vi "Panel.vi"(6 "Fiber Auto Collimation state data":refnum<class "Fiber Auto Collimation state data.lvclass">, 7 "Station config":refnum<class "Station config.lvclass">, 8 "error in":errorcluster, 11 "Fiber Auto Collimation configuration panel in":refnum<class "Fiber Auto Collimation configuration panel.lvclass">) -> (0 "error out":errorcluster, 3 "Fiber Auto Collimation configuration panel out":refnum<class "Fiber Auto Collimation configuration panel.lvclass">)   [LabVIEW 2018, in "Fiber Auto Collimation configuration panel.lvclass"]
doc: "This is the configuration panel. It is designed both as a starter location for all station administration controls and also to potentially be used as a template for copying to start off other Panel classes used on stations as well."
uses:
  Fiber Auto Collimation configuration panel.lvclass
  C:/LabVIEW Code/Fiber Auto Collimation/Source/Panels/Fiber Auto Collimation panel.lvclass
  State data/Fiber Auto Collimation state data.lvclass
  <userlib>/Recipe/Station Config/Station config.lvclass
  State data/Tracked state data.ctl
  State data/Fiber Auto Collimation state data.lvclass/Fiber Auto Collimation state data.ctl
  403c9101-8a94-4915-b1d2-c2bcb50c0ac3.vi
  14963872-09c7-484d-8f8b-814a5689ce7f.vi
  f712ade7-1d53-4238-a979-a732add69fae.vi
  403c9101-8a94-4915-b1d2-c2bcb50c0ac3.vi/f33612d2-cbd2-4a12-8b29-77b7af87b990.vi
  <userlib>/nLight Tidbits/Misc/Convert True to Enabled.vi
  <userlib>/nLight Error Handling/Log any errors.vi
  References/Obtain control updates queue.vi
  Misc SubVIs/Get control name.vi
  <userlib>/nLight Error Handling/Merge errors no loss.vi
  <userlib>/Recipe/Test Recipe classes/Test Recipe.lvclass
  ee343da0-43c2-4897-a8b1-c706a9c51c79.vi
  a23b397d-d5c1-4275-a046-494f1c6e56ee.vi
  References/Fiber Auto Collimation References.lvclass
  Fiber Auto Collimation panel.lvclass
panel:
  out "Loaded test recipe name":string
  in  "Upload test recipe":bool
  in  "Edit test recipe":bool
  in  "Edit test recipe keys":bool
  in  "Basic station config":bool
  in  "Edit station config keys":bool
  in  "Configure instruments":bool
  in  "Upload station config":bool
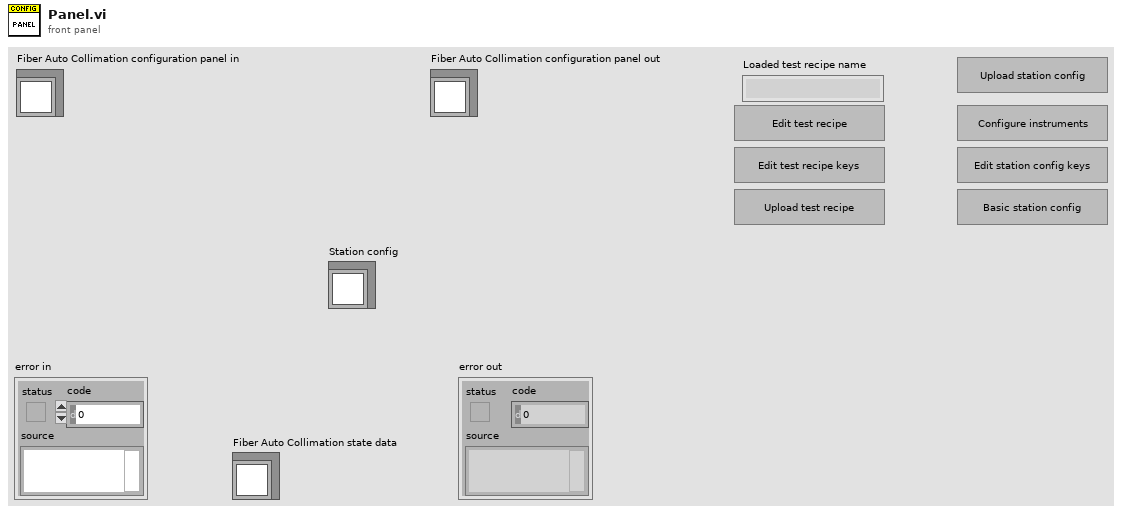
[diagram p1: front panel]
types:
  T1 = typedef "Fiber Auto Collimation state data.lvclass/Tracked state data.ctl" = enum16{"No update", "Permission level", "Username", "Test running", "DUT Serial", "Test status", "MOM Lot", "Loaded test recipe", "Model case running", "Station status", "BV data", "Defect Identify data", "Axis Position data", "Fiber Ass PN", "Operator", "RunTime", "VBAI", "Steps Cycle Time"}
  T2 = cluster{"事件注册引用句柄":refnum<event-registration>, "事件注册引用句柄":refnum<event-registration>}
  T3 = enum8{"Enabled", "Disabled", "Disabled and Grayed Out"}
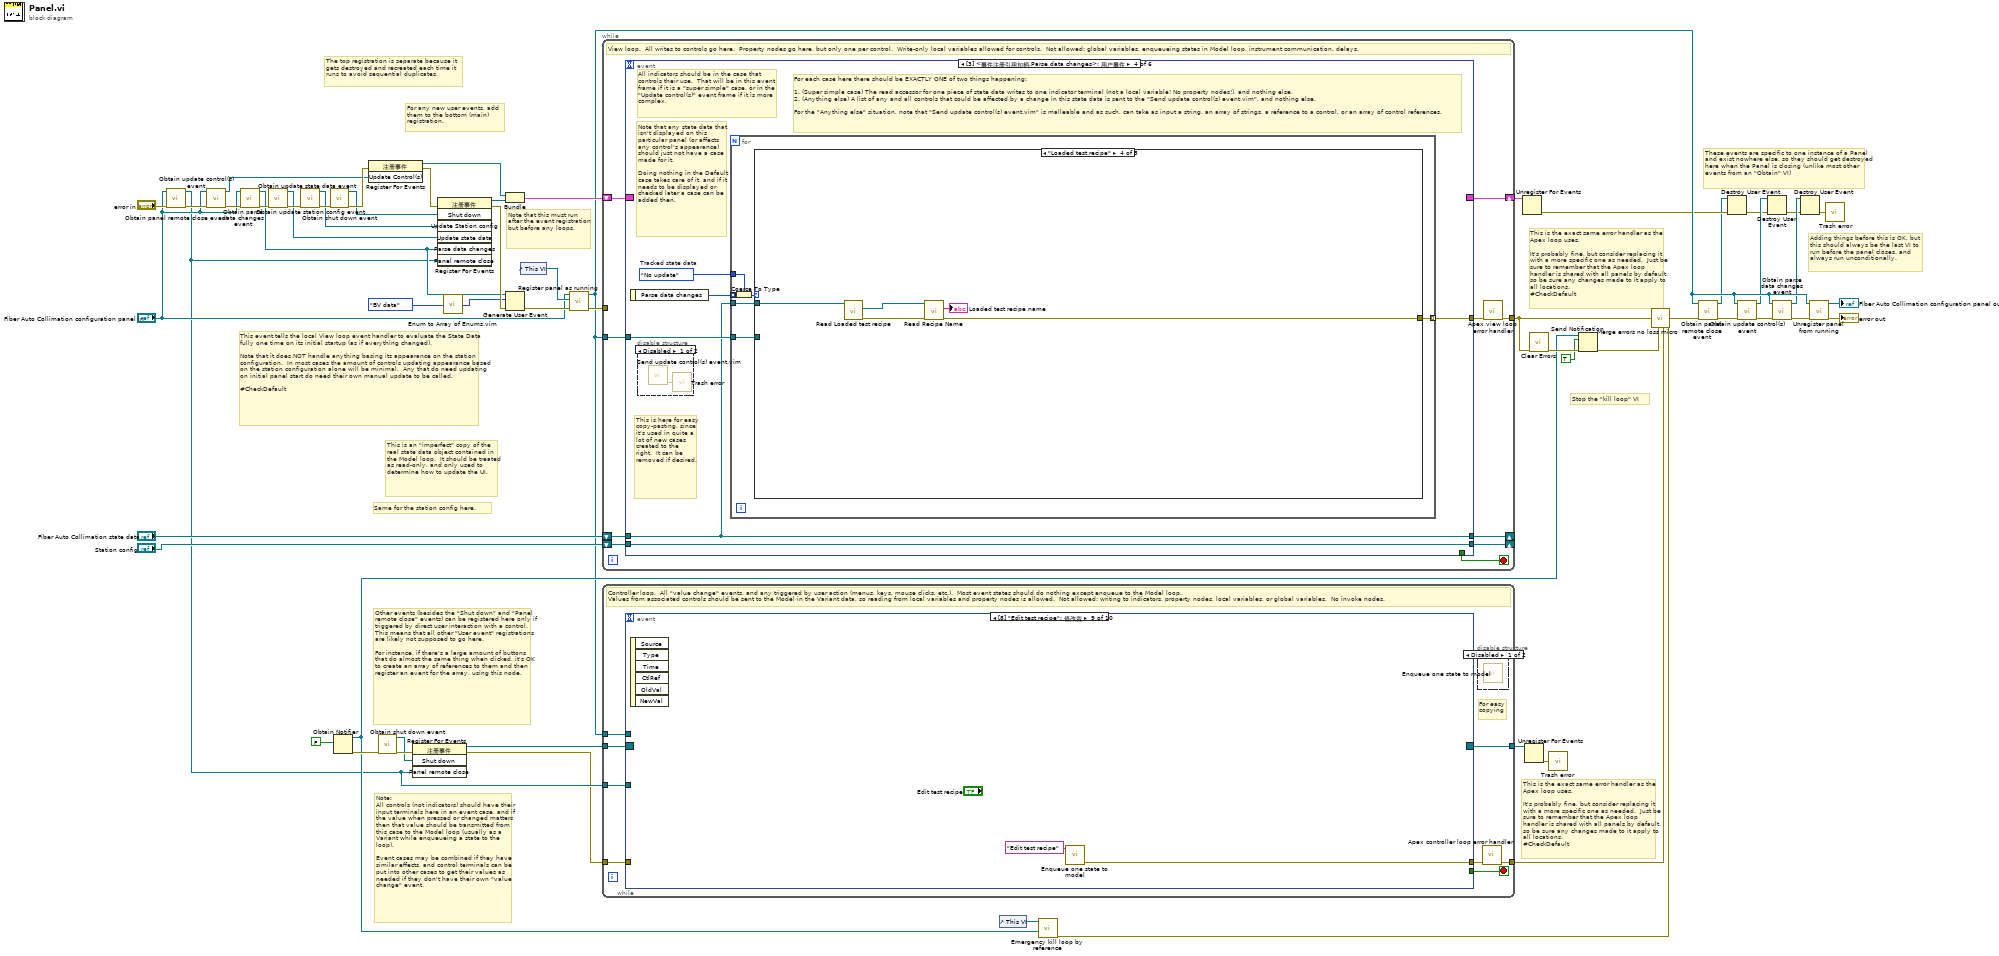
[diagram p0: block diagram]
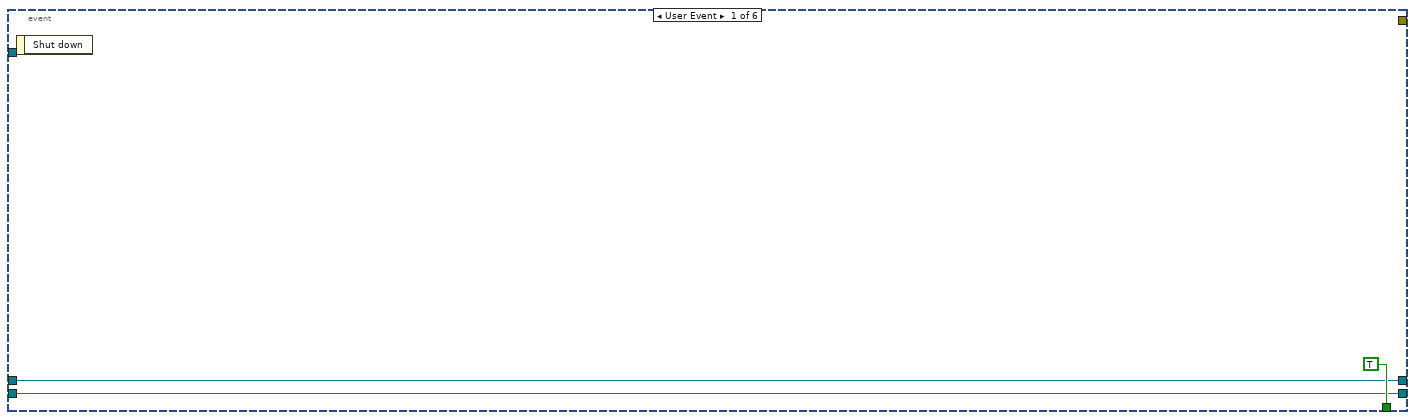
[diagram p2: hidden frame]
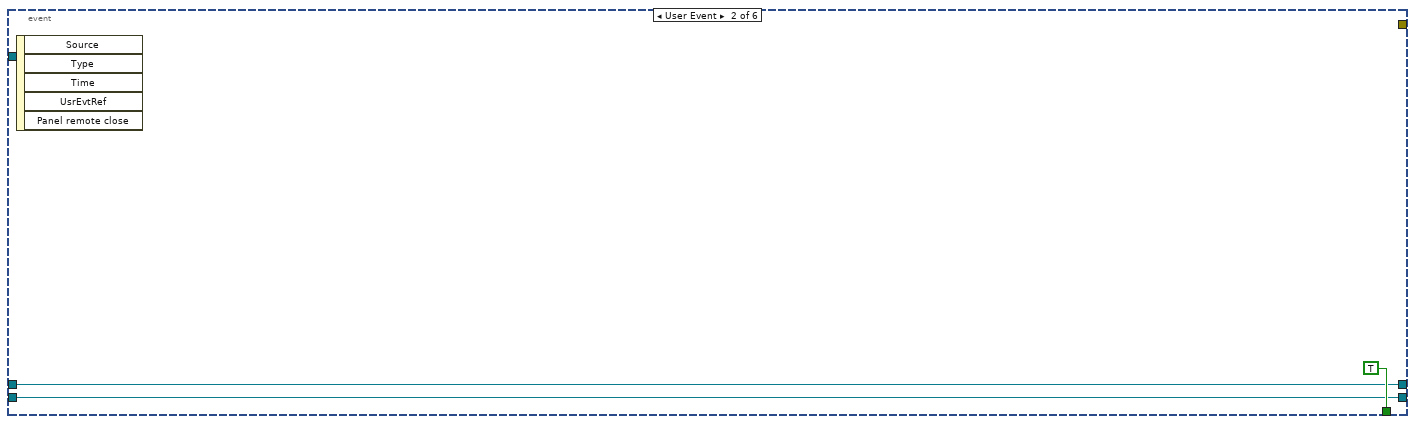
[diagram p3: hidden frame]
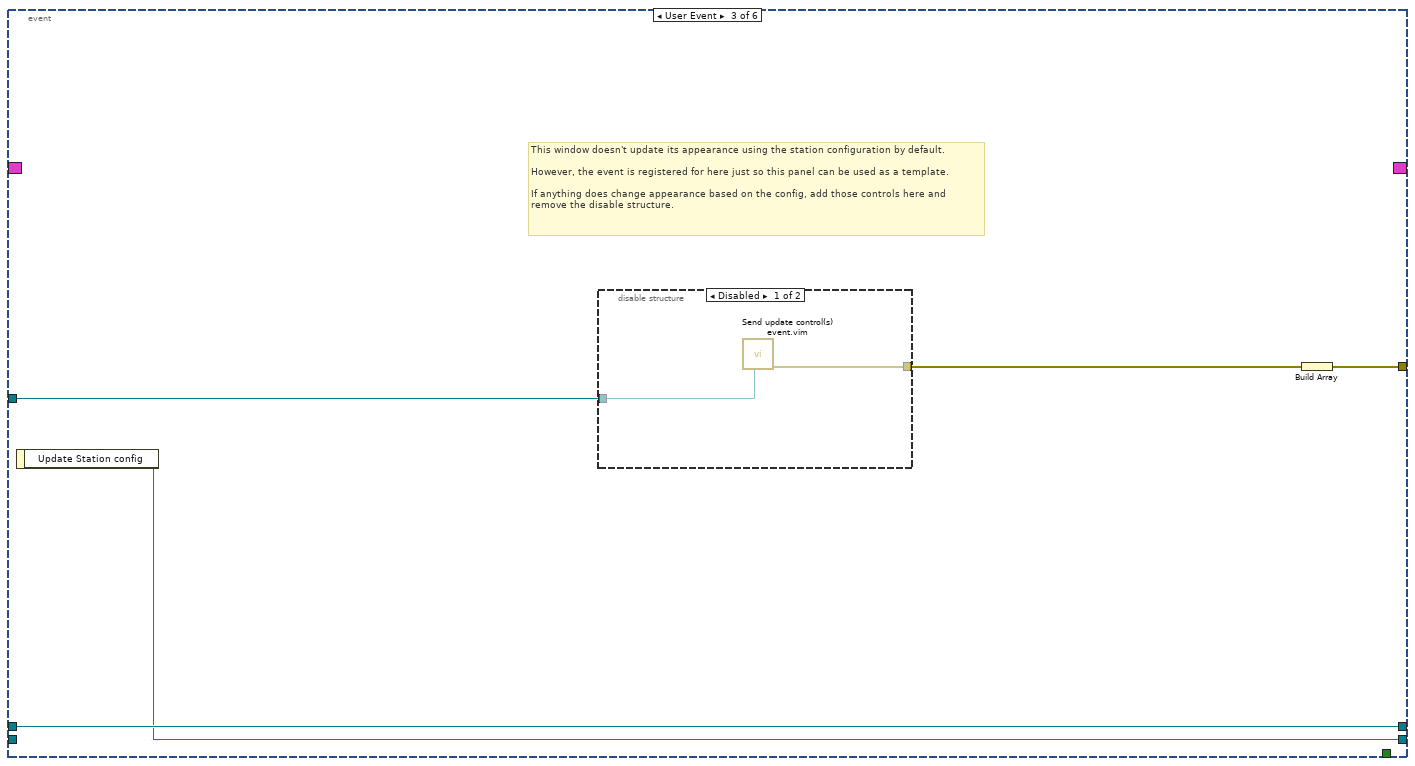
[diagram p4: hidden frame]
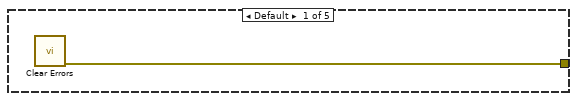
[diagram p7: hidden frame]
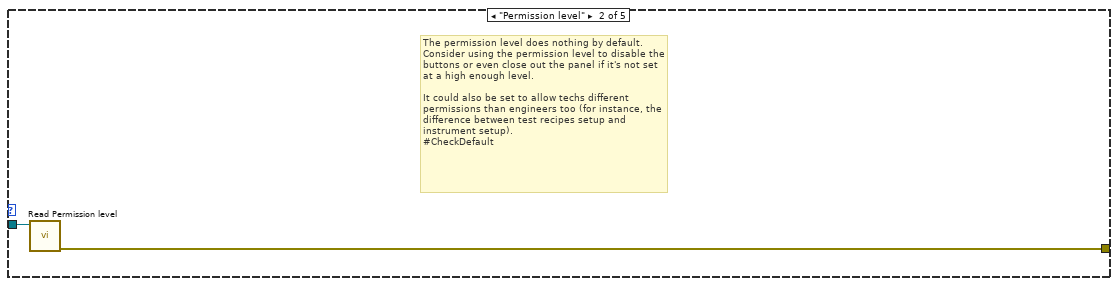
[diagram p8: hidden frame]
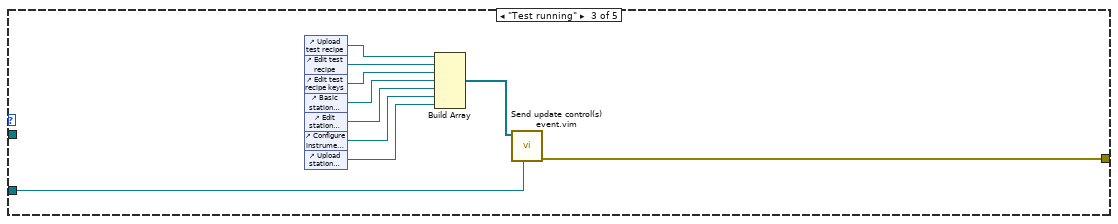
[diagram p9: hidden frame]
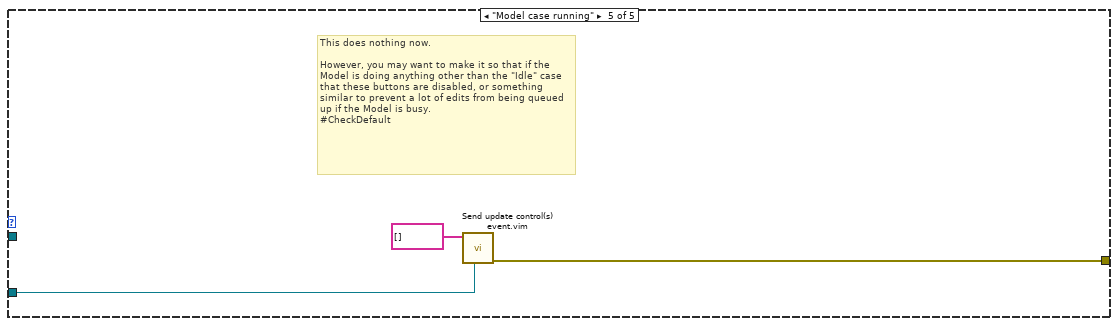
[diagram p10: hidden frame]
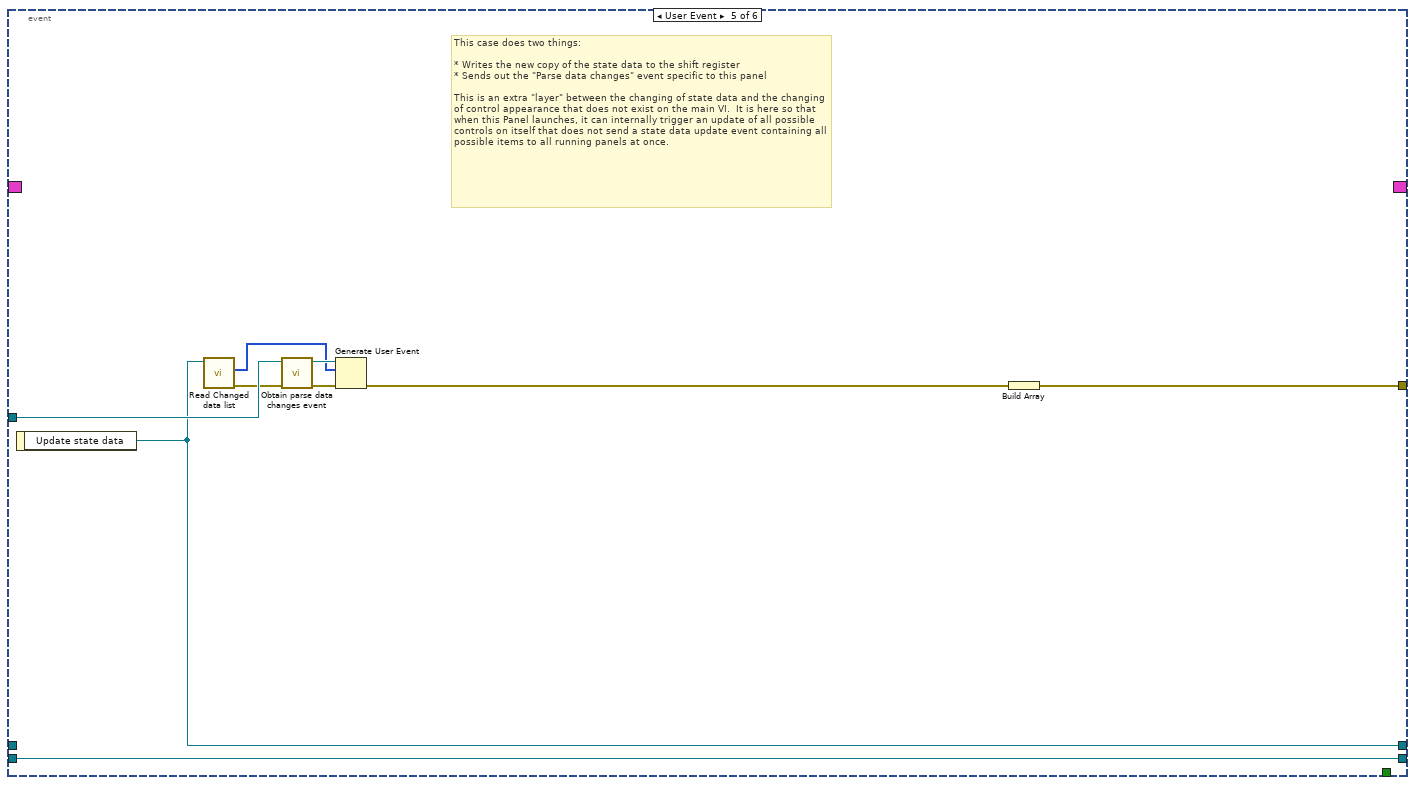
[diagram p11: hidden frame]
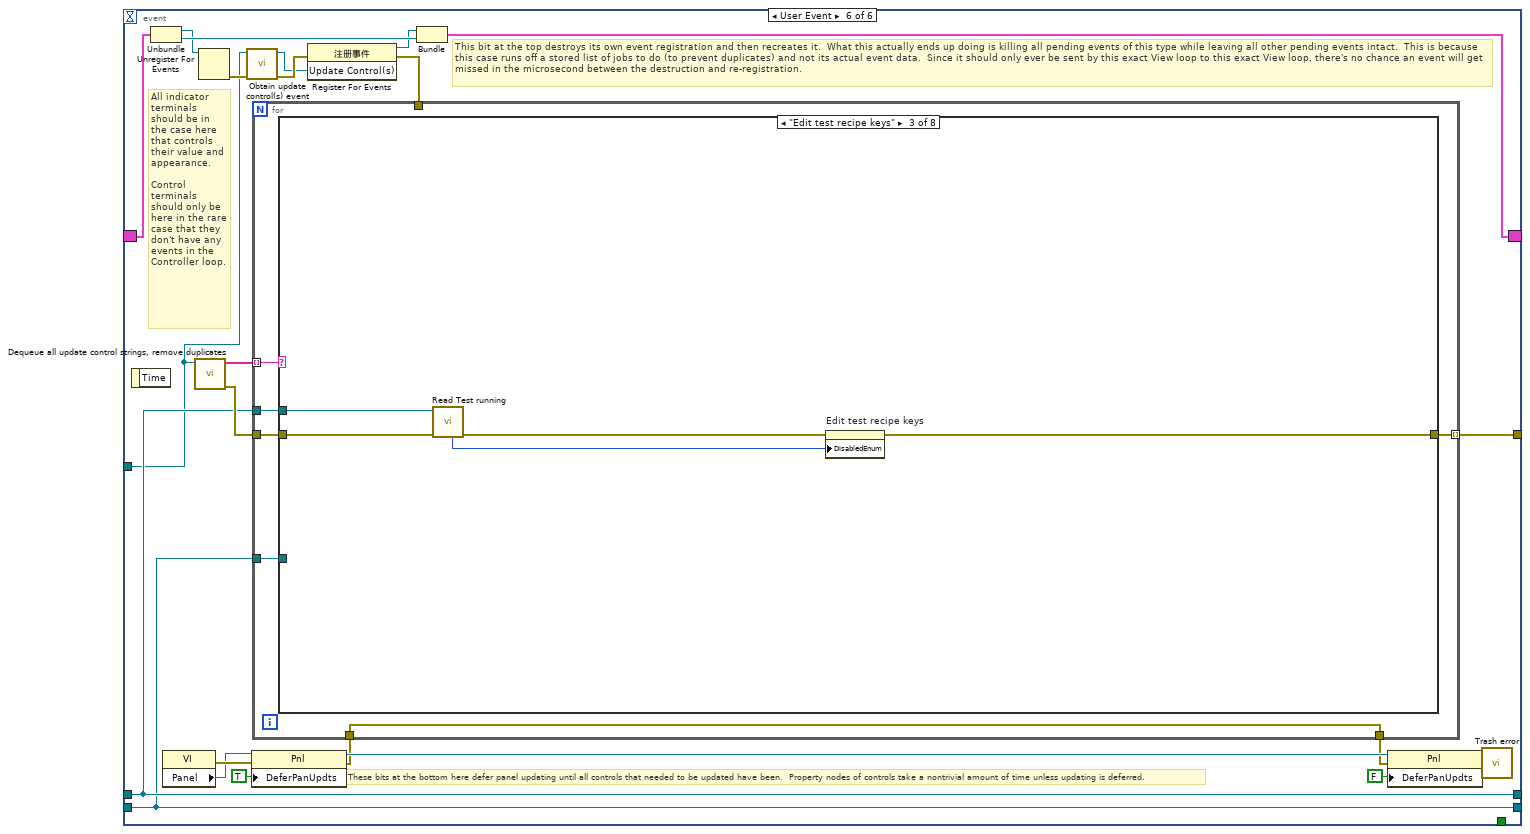
[diagram p12: hidden frame]
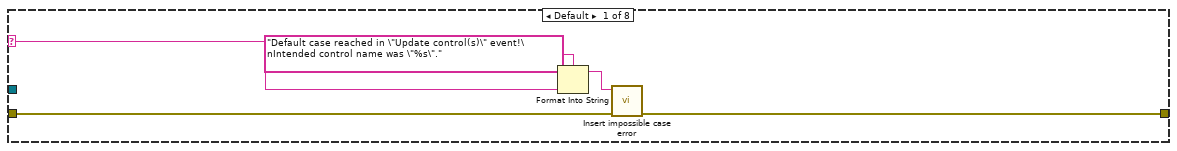
[diagram p13: hidden frame]
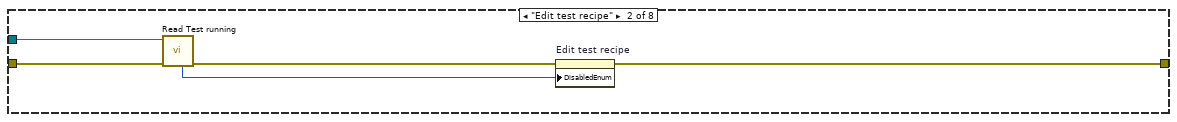
[diagram p14: hidden frame]
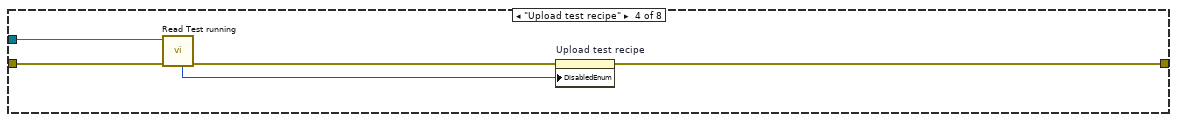
[diagram p15: hidden frame]
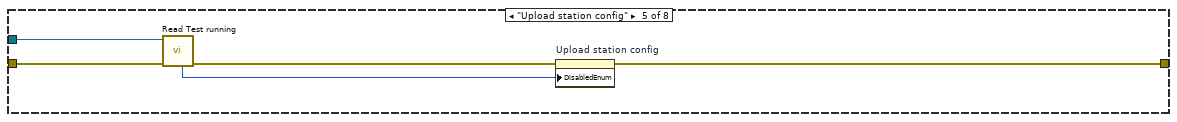
[diagram p16: hidden frame]
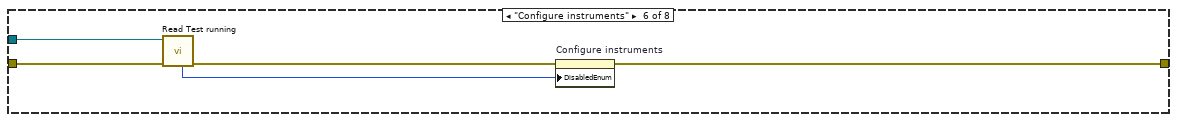
[diagram p17: hidden frame]
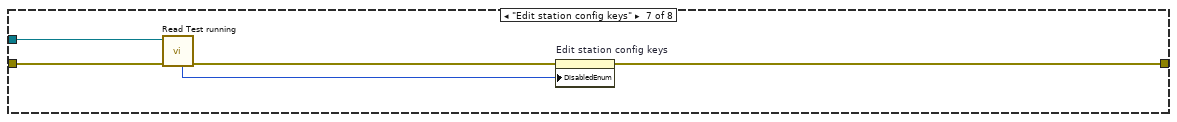
[diagram p18: hidden frame]
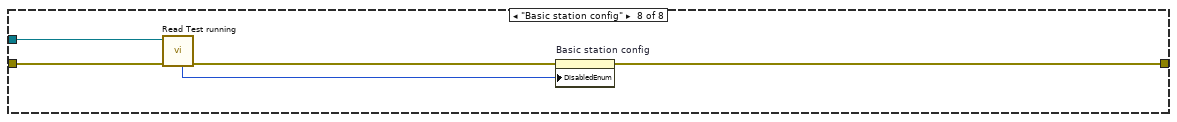
[diagram p19: hidden frame]
diagram:
  # "These events are specific to one instance of a Panel and exist nowhere else, so they should get destroyed here when the Panel is closing (unlike most other events from an \"Obtain\" VI)"
  # "This is the exact same error handler as the Apex loop uses.\n\nIt's probably fine, but consider replacing it with a more specific one as needed.  Just be sure to remember that the Apex loop handler is shared with all panels by default, so be sure any changes made to it apply to all locations.\n#CheckDefault"
  # "Note that this must run after the event registration but before any loops."
  # "This is the exact same error handler as the Apex loop uses.\n\nIt's probably fine, but consider replacing it with a more specific one as needed.  Just be sure to remember that the Apex loop handler is shared with all panels by default, so be sure any changes made to it apply to all locations.\n#CheckDefault"
  # "This event tells the local View loop event handler to evaluate the State Data fully one time on its initial startup (as if everything changed).\n\nNote that it does NOT handle anything basing its appearance on the station configuration.  In most cases the amount of controls updating appearance based on the station configuration alone will be minimal.  Any that do need updating on initial panel start do need their own manual update to be called.\n\n#CheckDefault"
  # "Adding things before this is OK, but this should always be the last VI to run before the panel closes, and always run unconditionally."
  # "Stop the \"kill loop\" VI"
  # "Same for the station config here."
  # "Note:\nAll controls (not indicators) should have their input terminals here in an event case, and if the value when pressed or changed matters then that value should be transmitted from this case to the Model loop (usually as a Variant while enqueueing a state to the loop).\n\nEvent cases may be combined if they have similar effects, and control terminals can be put into other cases to get their values as needed if they don't have their own \"value change\" event."
  # "Other events (besides the \"Shut down\" and \"Panel remote close\" events) can be registered here only if triggered by direct user interaction with a control.  This means that all other \"User event\" registrations are likely not supposed to go here.\n\nFor instance, if there's a large amount of buttons that do almost the same thing when clicked, it's OK to create an array of references to them and then register an event for the array, using this node."
  # "For any new user events, add them to the bottom (main) registration."
  # "The top registration is separate because it gets destroyed and recreated each time it runs to avoid sequential duplicates."
  # "This is an \"imperfect\" copy of the real state data object contained in the Model loop.  It should be treated as read-only, and only used to determine how to update the UI."
  n1 = call "Obtain panel remote close event.vi"("error in (no error)"="error in", "Fiber Auto Collimation panel"="Fiber Auto Collimation configuration panel in") -> ("error out"=w56:errorcluster, "Panel remote close"=w17:refnum<user-event>)  [unwired: 8 in]
  n2 = call "Obtain update control(s) event.vi"("error in (no error)"=w56, "Fiber Auto Collimation panel"="Fiber Auto Collimation configuration panel in") -> ("error out"=w27:errorcluster, "Update Control(s)"=w45:refnum<user-event>)  [unwired: 8 in]
  n3 = call "Obtain parse data changes event.vi"("error in (no error)"=w27, "Fiber Auto Collimation panel"="Fiber Auto Collimation configuration panel in") -> ("error out"=w26:errorcluster, "Parse data changes"=w24:refnum<user-event>)  [unwired: 8 in]
  n4 = call "Obtain update state data event.vi"("error in (no error)"=w26) -> ("error out"=w54:errorcluster, "Update state data"=w47:refnum<user-event>)  [unwired: 9 in]
  n5 = call "Obtain update station config event.vi"("error in"=w54) -> ("error out"=w49:errorcluster, "Update Station config"=w48:refnum<user-event>)  [unwired: 9 in]
  n6 = call "Obtain shut down event.vi"("error in (no error)"=w49) -> ("error out"=w57:errorcluster, "Shut down"=w53:refnum<user-event>)  [unwired: 9 in]
  n7 = Obtain Notifier(notification data type=FALSE) -> (notifier out=w38:refnum<notifier>, error out=w41:errorcluster)  [unwired: 3 in, 1 out]
  n8 = register-events(error in=w57, w45) -> (reference out=w44:refnum<event-registration>, error out=w32:errorcluster)  [unwired: 1 in]
  n9 = call "Obtain shut down event.vi"("error in (no error)"=w41) -> ("error out"=w52:errorcluster, "Shut down"=w51:refnum<user-event>)  [unwired: 9 in]
  n10 = register-events(error in=w52, w51, w17) -> (reference out=w50:refnum<event-registration>, error out=w1:errorcluster)  [unwired: 1 in]
  n11 = register-events(error in=w32, w53, w48, w47, w24, w17) -> (reference out=w46:refnum<event-registration>, error out=w55:errorcluster)  [unwired: 1 in]
  n12 = call "Enum to Array of Enums.vim"("enum"=Tracked_state_data."BV data" ("Tracked state data")) -> ("array of enums"=w23:T1[])
  n13 = Bundle("事件注册引用句柄"=w44, "事件注册引用句柄"=w46) -> (w43:T2)  [unwired: 1 in]
  n14 = Generate User Event(user event=w24, event data cluster=w23, error in=w55) -> (error out=w21:errorcluster)  [unwired: 1 in, 1 out]
  n15 = control-ref of="This VI"() -> (w31:refnum<vi>)
  n16 = call "Register panel as running.vi"("error in (no error)"=w21, "\"This VI\" reference from current panel"=w31, "Fiber Auto Collimation panel in"="Fiber Auto Collimation configuration panel in") -> ("error out"=w22:errorcluster, "Fiber Auto Collimation panel out"=w10:refnum<class "Fiber Auto Collimation configuration panel.lvclass">)  [unwired: 7 in]
  n17 = while {
    tunnel: [w67] -> w34
    shift-right: [w63] -> _
    shift-left: "Fiber Auto Collimation state data" -> [w62]
    shift-right: [w61] -> w16
    shift-left: w43 -> [w66]
    shift-right: [w60] -> _
    shift-left: "Station config" -> [w59]
    tunnel: w10 -> [w58]
    tunnel: w22 -> [_]
    stop <- w64 stop-if-true
    # "View loop.  All writes to controls go here.  Property nodes go here, but only one per control.  Write-only local variables allowed for controls.  Not allowed: global variables, enqueueing states in Model loop, instrument communication, delays."
    n18 = event "View" shown="[3] <事件注册引用句柄.Parse data changes>: 用户事件" {
      selector: w66 -> [_ _ _ _ _ w146]
      dyn-events: [_ _ _ _ _ w139] -> w61
      timeout: _ -> [_ _ _ _ _ _]
      tunnel: [_ _ w75 w86 w120 w128] -> w65
      tunnel: [TRUE TRUE _ _ _ _] -> w64
      tunnel: [w69 w72 w78 w83 w117 w129] -> w63
      tunnel: w62 -> [w69 w72 w78 w83 _ w129]
      tunnel: [w68 w71 w77 w85 w123 w126] -> w60
      tunnel: w59 -> [w68 w71 _ w85 w123 w126]
      tunnel: w58 -> [_ _ w74 w84 w122 w125]
      event User Event {
        n19 = event-data() -> ()  [unwired: 1 in, 1 out]
      }
      event User Event {
        n20 = event-data() -> ()  [unwired: 1 in, 5 out]
      }
      event User Event {
        # "This window doesn't update its appearance using the station configuration by default.\n\nHowever, the event is registered for here just so this panel can be used as a template.\n\nIf anything does change appearance based on the config, add those controls here and  remove the disable structure."
        n21 = event-data() -> ("Update Station config"=w77:refnum<class "Station config.lvclass">)  [unwired: 1 in]
        n22 = disable-structure shown="Disabled" {
          disable-tunnel: [w80 _] -> w76
          disable-tunnel: w74 -> [w79 _]
          frame Disabled {
            n23 = call "Send update control(s) event.vim"("Fiber Auto Collimation panel"=w79) -> ("error out"=w80:errorcluster)  [unwired: 10 in]
          }
          frame Enabled {
          }
        }
        n24 = Build Array(w76) -> (w75:errorcluster[])
      }
      event User Event {
        w81 = Tracked_state_data."No update"  # Tracked state data
        # "Note that any state data that isn't displayed on this particular panel (or affects any control's appearance) should just not have a case made for it.  \n\nDoing nothing in the Default case takes care of it, and if it needs to be displayed or checked later a case can be added then."
        # "All indicators should be in the case that controls their use.  That will be in this event frame if it is a \"super simple\" case, or in the \"Update control(s)\" event frame if it is more complex."
        # "This is here for easy copy-pasting, since it's used in quite a lot of new cases created to the right.  It can be removed if desired."
        # "For each case here there should be EXACTLY ONE of two things happening:\n\n1. (Super simple case) The read accessor for one piece of state data writes to one indicator terminal (not a local variable! No property nodes!), and nothing else.\n2. (Anything else) A list of any and all controls that could be affected by a change in this state data is sent to the \"Send update control(s) event.vim\", and nothing else.\n\nFor the \"Anything else\" situation, note that \"Send update control(s) event.vim\" is malleable and as such, can take as input a string, an array of strings, a reference to a control, or an array of control references."
        n25 = event-data() -> ("Parse data changes"=w82:u16[])  [unwired: 1 in]
        n26 = disable-structure shown="Disabled" {
          frame Disabled {
            n27 = call "Send update control(s) event.vim"() -> ("error out"=w87:errorcluster)  [unwired: 11 in]
            n28 = call <userlib>:"Trash error.vi"("error in"=w87) -> ()  [unwired: 15 in]
          }
          frame Enabled {
          }
        }
        n29 = for {
          tunnel: w82 -> [w93] mode=indexing
          tunnel: w83 -> [w92]
          tunnel: [w91] -> w86 mode=indexing
          tunnel: w84 -> [w90]
          tunnel: w81 -> [w88]
          n30 = Coerce To Type(0:w93, 1:w88) -> (2:w89:T1)
          n31 = case shown="\"Loaded test recipe\"" w89 {
            tunnel: w92 -> [_ w96 _ w111 _]
            tunnel: [w94 w95 w106 w108 w114] -> w91
            tunnel: w90 -> [_ _ w105 _ w112]
            frame Default {
              n32 = call <vilib>:"Clear Errors.vi"() -> ("error out"=w94:errorcluster)  [unwired: 6 in, 1 out]
            }
            frame "Permission level" {
              # "The permission level does nothing by default.  Consider using the permission level to disable the buttons or even close out the panel if it's not set at a high enough level.  \n\nIt could also be set to allow techs different permissions than engineers too (for instance, the difference between test recipes setup and instrument setup).\n#CheckDefault"
              n33 = call "Read Permission level.vi"("Fiber Auto Collimation state data in"=w96) -> ("error out"=w95:errorcluster)  [unwired: 8 in, 2 out]
            }
            frame "Test running" {
              n34 = control-ref of="Upload test recipe"() -> (w104:refnum<vi>)
              n35 = control-ref of="Edit test recipe"() -> (w103:refnum<vi>)
              n36 = control-ref of="Edit test recipe keys"() -> (w102:refnum<vi>)
              n37 = control-ref of="Basic station config"() -> (w101:refnum<vi>)
              n38 = control-ref of="Edit station config keys"() -> (w100:refnum<vi>)
              n39 = control-ref of="Configure instruments"() -> (w99:refnum<vi>)
              n40 = control-ref of="Upload station config"() -> (w98:refnum<vi>)
              n41 = Build Array(w104, w103, w102, w101, w100, w99, w98) -> (w97:refnum<vi>[])
              n42 = call "Send update control(s) event.vim"("Fiber Auto Collimation panel"=w105, "Control(s) [String or reference, can be array]"=w97) -> ("error out"=w106:errorcluster)  [unwired: 9 in]
            }
            frame "Loaded test recipe" {
              n43 = call "Read Loaded test recipe.vi"("Fiber Auto Collimation state data in"=w111) -> ("error out"=w109:errorcluster, "Loaded test recipe"=w110:refnum<class "Test Recipe.lvclass">)  [unwired: 8 in, 1 out]
              n44 = call-dynamic "Read Recipe Name.vi"("error in (no error)"=w109, "nLight Recipe in"=w110) -> ("error out"=w108:errorcluster, "Recipe Name"=→"Loaded test recipe name":string)  [unwired: 7 in, 1 out]
            }
            frame "Model case running" {
              # "This does nothing now.\n\nHowever, you may want to make it so that if the Model is doing anything other than the \"Idle\" case that these buttons are disabled, or something similar to prevent a lot of edits from being queued up if the Model is busy.\n#CheckDefault"
              n45 = call "Send update control(s) event.vim"("Fiber Auto Collimation panel"=w112, "Control(s) [String or reference, can be array]"=string[] []) -> ("error out"=w114:errorcluster)  [unwired: 9 in]
            }
          }
        }
      }
      event User Event {
        # "This case does two things:\n\n* Writes the new copy of the state data to the shift register\n* Sends out the \"Parse data changes\" event specific to this panel\n\nThis is an extra \"layer\" between the changing of state data and the changing of control appearance that does not exist on the main VI.  It is here so that when this Panel launches, it can internally trigger an update of all possible controls on itself that does not send a state data update event containing all possible items to all running panels at once."
        n46 = event-data() -> ("Update state data"=w117:refnum<class "Fiber Auto Collimation state data.lvclass">)  [unwired: 1 in]
        n47 = call "Read Changed data list.vi"("Fiber Auto Collimation state data in"=w117) -> ("error out"=w116:errorcluster, "Changed data list"=w115:T1[])  [unwired: 8 in, 1 out]
        n48 = call "Obtain parse data changes event.vi"("error in (no error)"=w116, "Fiber Auto Collimation panel"=w122) -> ("error out"=w121:errorcluster, "Parse data changes"=w118:refnum<user-event>)  [unwired: 8 in]
        n49 = Generate User Event(user event=w118, event data cluster=w115, error in=w121) -> (error out=w119:errorcluster)  [unwired: 1 in, 1 out]
        n50 = Build Array(w119) -> (w120:errorcluster[])
      }
      event User Event {
        # "All indicator terminals should be in the case here that controls their value and appearance.\n\nControl terminals should only be here in the rare case that they don't have any events in the Controller loop."
        # "These bits at the bottom here defer panel updating until all controls that needed to be updated have been.  Property nodes of controls take a nontrivial amount of time unless updating is deferred."
        # "This bit at the top destroys its own event registration and then recreates it.  What this actually ends up doing is killing all pending events of this type while leaving all other pending events intact.  This is because this case runs off a stored list of jobs to do (to prevent duplicates) and not its actual event data.  Since it should only ever be sent by this exact View loop to this exact View loop, there's no chance an event will get missed in the microsecond between the destruction and re-registration."
        n51 = event-data() -> ()  [unwired: 1 in, 1 out]
        n52 = Unbundle(w146) -> ("事件注册引用句柄"=w144:refnum<event-registration>, "事件注册引用句柄"=w145:refnum<event-registration>)
        n53 = property class="VI"() -> (error out=w138:errorcluster, "Panel"=w136:refnum<vi>)  [unwired: 2 in, 1 out]
        n54 = call "Dequeue all update control strings, remove duplicates.vi"("Fiber Auto Collimation panel"=w125) -> ("error out"=w133:errorcluster, "Controls to update"=w132:string[])  [unwired: 9 in]
        n55 = Unregister For Events(event registration refnum=w144) -> (error out=w143:errorcluster)  [unwired: 1 in]
        n56 = call "Obtain update control(s) event.vi"("error in (no error)"=w143, "Fiber Auto Collimation panel"=w125) -> ("error out"=w142:errorcluster, "Update Control(s)"=w141:refnum<user-event>)  [unwired: 8 in]
        n57 = property class="Pnl"(reference=w136, error in=w138, "DeferPanUpdts"=TRUE ("Defer Panel Updates")) -> (reference out=w134:refnum<vi>, error out=w131:errorcluster)
        n58 = register-events(error in=w142, w141) -> (reference out=w140:refnum<event-registration>, error out=w127:errorcluster)  [unwired: 1 in]
        n59 = for {
          tunnel: w133 -> [w151]
          tunnel: w132 -> [w152] mode=indexing
          tunnel: [w150] -> w128 mode=indexing
          tunnel: w131 -> [w149]
          tunnel: [w149] -> w130
          tunnel: w129 -> [w148]
          tunnel: w127 -> [_]
          tunnel: w126 -> [w147]
          n60 = case shown="\"Edit test recipe keys\"" w152 {
            selector: w152 -> [w155 _ _ _ _ _ _ _]
            tunnel: w151 -> [w154 w162 w167 w172 w177 w182 w187 w192]
            tunnel: [w153 w158 w163 w168 w173 w178 w183 w188] -> w150
            tunnel: w148 -> [_ w161 w166 w171 w176 w181 w186 w191]
            tunnel: w147 -> [_ _ _ _ _ _ _ _]
            frame Default {
              n61 = Format Into String(format string="Default case reached in \"Update control(s)\" event!\nIntended control name was \"%s\".", w155) -> (resulting string=w156:string)  [unwired: 2 in, 1 out]
              n62 = call <userlib>:"Insert impossible case error.vi"("error in (no error)"=w154, "Optional extra info"=w156) -> ("error out"=w153:errorcluster)  [unwired: 9 in]
            }
            frame "Edit test recipe" {
              n63 = call "Read Test running.vi"("error in (no error)"=w162, "Fiber Auto Collimation state data in"=w161) -> ("error out"=w159:errorcluster, "Disable control(s) when test is running"=w160:T3)  [unwired: 6 in, 2 out]
              n64 = property on="Edit test recipe" class="Bool"(error in=w159, "DisabledEnum"=w160) -> (error out=w158:errorcluster)  [unwired: 1 in, 1 out]
            }
            frame "Edit test recipe keys" {
              n65 = call "Read Test running.vi"("error in (no error)"=w167, "Fiber Auto Collimation state data in"=w166) -> ("error out"=w164:errorcluster, "Disable control(s) when test is running"=w165:T3)  [unwired: 6 in, 2 out]
              n66 = property on="Edit test recipe keys" class="Bool"(error in=w164, "DisabledEnum"=w165) -> (error out=w163:errorcluster)  [unwired: 1 in, 1 out]
            }
            frame "Upload test recipe" {
              n67 = call "Read Test running.vi"("error in (no error)"=w172, "Fiber Auto Collimation state data in"=w171) -> ("error out"=w169:errorcluster, "Disable control(s) when test is running"=w170:T3)  [unwired: 6 in, 2 out]
              n68 = property on="Upload test recipe" class="Bool"(error in=w169, "DisabledEnum"=w170) -> (error out=w168:errorcluster)  [unwired: 1 in, 1 out]
            }
            frame "Upload station config" {
              n69 = call "Read Test running.vi"("error in (no error)"=w177, "Fiber Auto Collimation state data in"=w176) -> ("error out"=w174:errorcluster, "Disable control(s) when test is running"=w175:T3)  [unwired: 6 in, 2 out]
              n70 = property on="Upload station config" class="Bool"(error in=w174, "DisabledEnum"=w175) -> (error out=w173:errorcluster)  [unwired: 1 in, 1 out]
            }
            frame "Configure instruments" {
              n71 = call "Read Test running.vi"("error in (no error)"=w182, "Fiber Auto Collimation state data in"=w181) -> ("error out"=w179:errorcluster, "Disable control(s) when test is running"=w180:T3)  [unwired: 6 in, 2 out]
              n72 = property on="Configure instruments" class="Bool"(error in=w179, "DisabledEnum"=w180) -> (error out=w178:errorcluster)  [unwired: 1 in, 1 out]
            }
            frame "Edit station config keys" {
              n73 = call "Read Test running.vi"("error in (no error)"=w187, "Fiber Auto Collimation state data in"=w186) -> ("error out"=w184:errorcluster, "Disable control(s) when test is running"=w185:T3)  [unwired: 6 in, 2 out]
              n74 = property on="Edit station config keys" class="Bool"(error in=w184, "DisabledEnum"=w185) -> (error out=w183:errorcluster)  [unwired: 1 in, 1 out]
            }
            frame "Basic station config" {
              n75 = call "Read Test running.vi"("error in (no error)"=w192, "Fiber Auto Collimation state data in"=w191) -> ("error out"=w189:errorcluster, "Disable control(s) when test is running"=w190:T3)  [unwired: 6 in, 2 out]
              n76 = property on="Basic station config" class="Bool"(error in=w189, "DisabledEnum"=w190) -> (error out=w188:errorcluster)  [unwired: 1 in, 1 out]
            }
          }
        }
        n77 = Bundle("事件注册引用句柄"=w140, "事件注册引用句柄"=w145) -> (w139:T2)  [unwired: 1 in]
        n78 = property class="Pnl"(reference=w134, error in=w130, "DeferPanUpdts"=FALSE ("Defer Panel Updates")) -> (error out=w124:errorcluster)  [unwired: 1 out]
        n79 = call <userlib>:"Trash error.vi"("error in"=w124) -> ()  [unwired: 15 in]
      }
    }
    n80 = call "Apex view loop error handler.vi"("errors in"=w65) -> ("error out"=w67:errorcluster)  [unwired: 10 in]
  }
  n81 = while {
    tunnel: [w200] -> w28
    tunnel: w50 -> [w199]
    tunnel: w10 -> [w196]
    tunnel: w17 -> [w195]
    tunnel: [w194] -> w15
    tunnel: w1 -> [w193]
    stop <- w198 stop-if-true
    # "For easy copying"
    # "Controller loop.  All \"value change\" events, and any triggered by user action (menus, keys, mouse clicks, etc.).  Most event states should do nothing except enqueue to the Model loop.\nValues from associated controls should be sent to the Model in the Variant data, so reading from local variables and property nodes is allowed.  Not allowed: writing to indicators, property nodes, local variables, or global variables.  No invoke nodes."
    n82 = event "Controller [Value change events go here]" shown="[8] \"Edit test recipe\": 值改变" {
      selector: w199 -> [_ _ _ _ _ _ _ _ _ _]
      dyn-events: [_ _ _ _ _ _ _ _ _ _] -> w194
      timeout: _ -> [_ _ _ _ _ _ _ _ _ _]
      tunnel: [TRUE TRUE _ _ _ _ _ _ _ _] -> w198
      tunnel: [w201 w203 w206 w210 w211 w213 w215 w217 w219 w222] -> w197
      tunnel: w196 -> [_ _ w207 _ _ _ _ _ _ _]
      tunnel: w195 -> [_ _ w208 _ _ _ _ _ _ _]
      tunnel: w193 -> [w201 _ w205 _ _ _ _ _ _ _]
      event User Event {
        n83 = event-data() -> ()  [unwired: 1 in, 5 out]
      }
      event User Event {
        n84 = event-data() -> ()  [unwired: 1 in, 5 out]
        n85 = call <vilib>:"Clear Errors.vi"() -> ("error out"=w203:errorcluster)  [unwired: 6 in, 1 out]
      }
      event Panel Close {
        # "This panel hides itself as soon as someone hits the \"X\" in the corner, but the code is still running until the \"Panel remote close\" event is triggered, ending both event loops on the page.\n\nNormally this is fine, but if any state data needs to change as a result of this panel closing make sure any instructions needed to do that are enqueued here as well. \n#CheckDefault"
        n86 = event-data() -> ()  [unwired: 1 in, 4 out]
        n87 = Generate User Event(user event=w208, event data cluster=w207, error in=w205) -> (error out=w206:errorcluster)  [unwired: 1 in, 1 out]
      }
      event "Upload station config": Value Change {
        n88 = event-data() -> ()  [unwired: 1 in, 6 out]
        n89 = call "Enqueue one state to model.vi"("Enqueued state"="Upload station config") -> ("error out"=w210:errorcluster)  [unwired: 10 in]
      }
      event "Configure instruments": Value Change {
        n90 = event-data() -> ()  [unwired: 1 in, 6 out]
        n91 = call "Enqueue one state to model.vi"("Enqueued state"="Configure instruments") -> ("error out"=w211:errorcluster)  [unwired: 10 in]
      }
      event "Edit station config keys": Value Change {
        n92 = event-data() -> ()  [unwired: 1 in, 6 out]
        n93 = call "Enqueue one state to model.vi"("Enqueued state"="Edit station config keys") -> ("error out"=w213:errorcluster)  [unwired: 10 in]
      }
      event "Basic station config": Value Change {
        n94 = event-data() -> ()  [unwired: 1 in, 6 out]
        n95 = call "Enqueue one state to model.vi"("Enqueued state"="Basic station config") -> ("error out"=w215:errorcluster)  [unwired: 10 in]
      }
      event "Edit test recipe keys": Value Change {
        n96 = event-data() -> ()  [unwired: 1 in, 6 out]
        n97 = call "Enqueue one state to model.vi"("Enqueued state"="Edit test recipe keys") -> ("error out"=w217:errorcluster)  [unwired: 10 in]
      }
      event "Edit test recipe": Value Change {
        n98 = event-data() -> ()  [unwired: 1 in, 6 out]
        n99 = call "Enqueue one state to model.vi"("Enqueued state"="Edit test recipe") -> ("error out"=w219:errorcluster)  [unwired: 10 in]
      }
      event "Upload test recipe": Value Change {
        n100 = event-data() -> ()  [unwired: 1 in, 6 out]
        n101 = call "Enqueue one state to model.vi"("Enqueued state"="Upload test recipe") -> ("error out"=w222:errorcluster)  [unwired: 10 in]
      }
    }
    n102 = disable-structure shown="Disabled" {
      frame Disabled {
        n103 = call "Enqueue one state to model.vi"() -> ()  [unwired: 11 in, 1 out]
      }
      frame Enabled {
      }
    }
    n104 = call "Apex controller loop error handler.vi"("error in"=w197) -> ("error out"=w200:errorcluster)  [unwired: 10 in]
  }
  n105 = control-ref of="This VI"() -> (w40:refnum<vi>)
  n106 = call "Emergency kill loop by reference.vi"("Quit early notifier"=w38, "VI reference in"=w40) -> ("error out"=w29:errorcluster)  [unwired: 9 in]
  n107 = Unregister For Events(event registration refnum=w16) -> (error out=w9:errorcluster)  [unwired: 1 in]
  n108 = Unregister For Events(event registration refnum=w15) -> (error out=w2:errorcluster)  [unwired: 1 in]
  n109 = call <vilib>:"Clear Errors.vi"("error in (no error)"=w34) -> ("error out"=w39:errorcluster)  [unwired: 5 in, 1 out]
  n110 = call <userlib>:"Trash error.vi"("error in"=w2) -> ()  [unwired: 15 in]
  n111 = Send Notification(notification=TRUE, notifier=w38, error in (no error)=w39) -> (error out=w30:errorcluster)  [unwired: 1 out]
  n112 = call <userlib>:"Merge errors no loss micro.vi"("error in (no error) 1"=w34, "error in (no error) 5"=w30, "error in (no error) 6"=w28, "error in (no error) 7"=w29) -> ("error out"=w14:errorcluster)  [unwired: 5 in]
  n113 = call "Obtain panel remote close event.vi"("error in (no error)"=w14, "Fiber Auto Collimation panel"=w10) -> ("error out"=w13:errorcluster, "Panel remote close"=w8:refnum<user-event>)  [unwired: 8 in]
  n114 = Destroy User Event(user event=w8, error in=w9) -> (error out=w5:errorcluster)
  n115 = call "Obtain update control(s) event.vi"("error in (no error)"=w13, "Fiber Auto Collimation panel"=w10) -> ("error out"=w12:errorcluster, "Update Control(s)"=w6:refnum<user-event>)  [unwired: 8 in]
  n116 = Destroy User Event(user event=w6, error in=w5) -> (error out=w4:errorcluster)
  n117 = call "Obtain parse data changes event.vi"("error in (no error)"=w12, "Fiber Auto Collimation panel"=w10) -> ("error out"=w11:errorcluster, "Parse data changes"=w7:refnum<user-event>)  [unwired: 8 in]
  n118 = Destroy User Event(user event=w7, error in=w4) -> (error out=w3:errorcluster)
  n119 = call "Unregister panel from running.vi"("error in (no error)"=w11, "Fiber Auto Collimation panel in"=w10) -> ("error out"=→"error out":errorcluster, "Fiber Auto Collimation panel out"=→"Fiber Auto Collimation configuration panel out":refnum<class "Fiber Auto Collimation configuration panel.lvclass">)  [unwired: 8 in]
  n120 = call <userlib>:"Trash error.vi"("error in"=w3) -> ()  [unwired: 15 in]
